vi "FP to PGSQL.vi"(0 "FP Data":sgl[](array[numeric]), 5 "MG Data":dbl[](array[numeric]), 7 "PT Data":dbl[](array[numeric]), 9 "FP Status Bits":u32[](array[numeric]), 11 "Mode":u16) -> ()   [LabVIEW 2019, in "FP-TC-Shared.lvclass"]
uses:
  FP-TC-Shared.lvclass
  FP-TC-Shared.lvclass/FP-TC-Shared.ctl
  <vilib>/Platform/browser.llb/Open URL in Default Browser (string).vi
  <userlib>/LevyLab/LV-Data/LV-Data.PG/LV-Data.PGSQL.lvclass
  <userlib>/LevyLab/LV-Data/LV-Data.PG/API/Write Variable (one-row).vi
panel:
  in  "error in (no error)":errorcluster
  out "error out":errorcluster
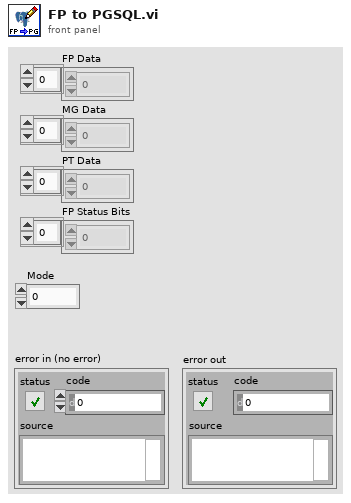
[diagram p1: front panel]
types:
  T1 = typedef "FP-TC-Shared.lvclass/LC Type--Enum.ctl" = enum16{"CF.TC", "CF.TC.Z", "CF.FP", "MNK.TC", "MNK.TC.Z", "MNK.FP"}
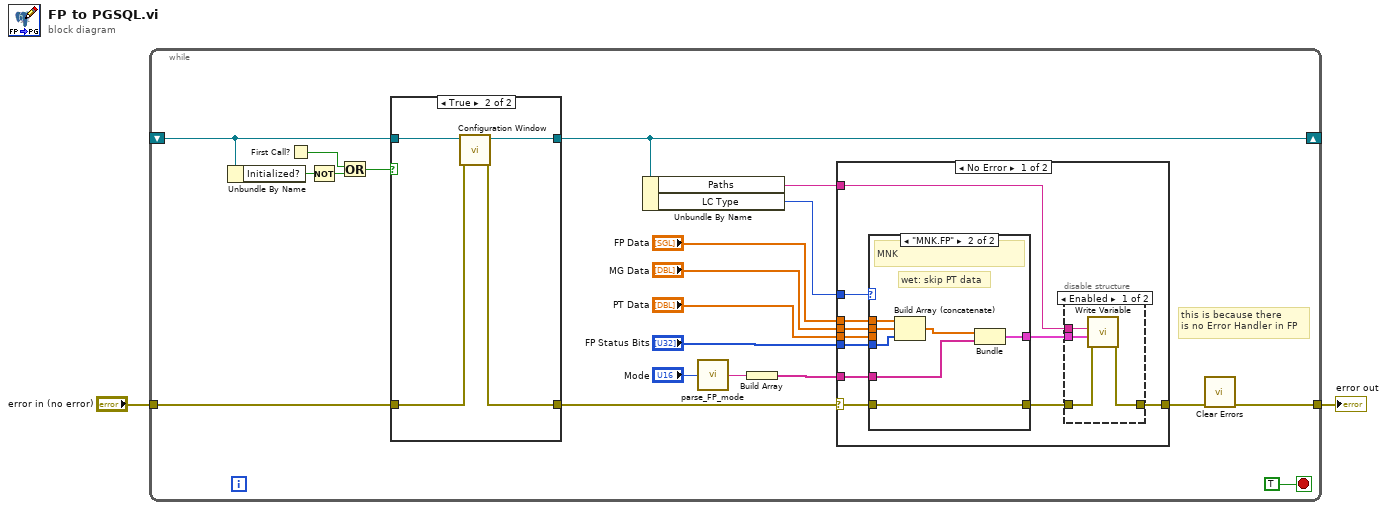
[diagram p0: block diagram]
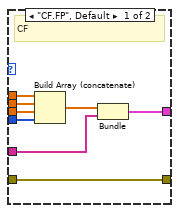
[diagram p4: hidden frame]
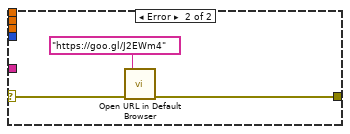
[diagram p5: hidden frame]
diagram:
  n1 = while {
    tunnel: [w19] -> w2
    tunnel: "error in (no error)" -> [w7]
    shift-right: [w5] -> _
    shift-left: _ -> [w6]
    stop <- TRUE stop-if-true
    # "this is because there\nis no Error Handler in FP"
    n2 = Unbundle By Name(w6) -> ("Initialized?"=w10:bool)
    n3 = First Call?() -> (First Call?: T/F=w12:bool)
    n4 = Not(x=w10) -> (.not. x?=w11:bool)
    n5 = Or(x=w12, y=w11) -> (x .or. y?=w9:bool)
    n6 = case shown="True" w9 {
      tunnel: [w24 w28] -> w5
      tunnel: w6 -> [w24 w25]
      tunnel: [w23 w26] -> w8
      tunnel: w7 -> [w23 w27]
      frame False {
      }
      frame True {
        n7 = call-dynamic "Configuration Window.vi"("error in (no error)"=w27, "FP-TC-Shared"=w25) -> ("error out"=w26:errorcluster, "FP-TC-Shared out"=w28:refnum<class "FP-TC-Shared.lvclass">)  [unwired: 8 in]
      }
    }
    n8 = Unbundle By Name(w5) -> ("Paths"=w3:string, "LC Type"=w4:T1)
    n9 = call "parse_FP_mode.vi"("line index"="Mode") -> ("output string"=w21:string)
    n10 = Build Array(w21) -> (w22:string[])
    n11 = case shown="No Error" w8 {
      selector: w8 -> [w34 w61]
      tunnel: w22 -> [w39 _]
      tunnel: "PT Data" -> [w38 _]
      tunnel: "MG Data" -> [w37 _]
      tunnel: "FP Data" -> [w36 _]
      tunnel: "FP Status Bits" -> [w35 _]
      tunnel: [w30 w60] -> w20
      tunnel: w4 -> [w33 _]
      tunnel: w3 -> [w29 _]
      frame No Error {
        n12 = case shown="\"MNK.FP\"" w33 {
          tunnel: w36 -> [w51 w58]
          tunnel: w37 -> [w50 w57]
          tunnel: w38 -> [w49 _]
          tunnel: w39 -> [w44 w54]
          tunnel: w35 -> [w48 w56]
          tunnel: w34 -> [w45 w52]
          tunnel: [w45 w52] -> w31
          tunnel: [w46 w53] -> w32
          frame "CF.FP", Default {
            # "CF"
            n13 = Build Array (concatenate)(w51, w50, w49, w48) -> (w47:dbl[])
            n14 = Bundle(w47, w44) -> (w46:cluster{dbl[], string[]})  [unwired: 1 in]
          }
          frame "MNK.FP" {
            # "wet: skip PT data"
            # "MNK"
            n15 = Build Array (concatenate)(w58, w57, w56) -> (w55:dbl[])
            n16 = Bundle(w55, w54) -> (w53:cluster{dbl[], string[]})  [unwired: 1 in]
          }
        }
        n17 = disable-structure shown="Enabled" {
          disable-tunnel: w32 -> [w43 _]
          disable-tunnel: w31 -> [w42 _]
          disable-tunnel: [w41 _] -> w30
          disable-tunnel: w29 -> [w40 _]
          frame Enabled {
            n18 = call-poly <userlib>:"Write Variable.vi"("error in (no error)"=w42, "Data"=w43, "variable"=w40) -> ("error out"=w41:errorcluster)  [unwired: 5 in, 3 out]
          }
          frame Disabled {
          }
        }
      }
      frame Error {
        n19 = call-poly <vilib>:"Open URL in Default Browser.vi"("error in (no error)"=w61, "URL"="https://goo.gl/J2EWm4") -> ("error out"=w60:errorcluster)  [unwired: 4 in, 1 out]
      }
    }
    n20 = call <vilib>:"Clear Errors.vi"("error in (no error)"=w20) -> ("error out"=w19:errorcluster)  [unwired: 5 in, 1 out]
  }
  "error out" <- w2
